vi "MS Updater.vi"(1 "Conveyer Belt Info":T1) -> (0 "Conveyer Belt Info out":T1)   [LabVIEW 2012]
uses:
  Cannon/Cannon Global Data.vi
panel:
  # "s"
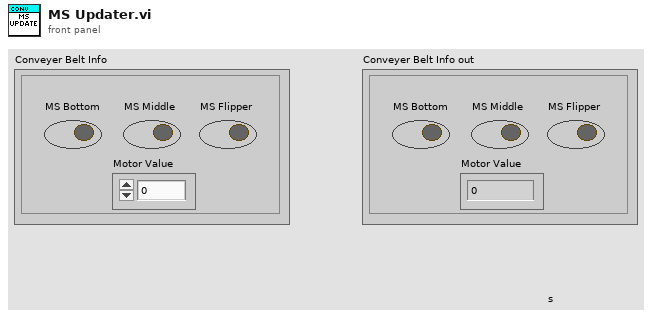
[diagram p1: front panel]
types:
  T1 = cluster{"MS Bottom":bool, "MS Middle":bool, "MS Flipper":bool, "Motor Value":dbl}
  T2 = cluster{"RPM":dbl, "Trigger":bool, "Angle Axis":dbl, "Angle":dbl, "Throttle":dbl, "Slow Angle Change?":bool, "Angle Change?":bool}
  T3 = typedef "WPI_DigitalInputDevRef.ctl" = cluster{"DevStatus":errorcluster, "DIO Channel":T4, "Digital Module":T5}
  T4 = typedef "FPGA_DIOChannel.ctl" = enum8{"DIO 1", "DIO 2", "DIO 3", "DIO 4", "DIO 5", "DIO 6", "DIO 7", "DIO 8", "DIO 9", "DIO 10", "DIO 11", "DIO 12", "DIO 13", "DIO 14", "Invalid"}
  T5 = typedef "FPGA_TypedefDigitalModule.ctl" = enum16{"Digital Module 1", "Digital Module 2"}
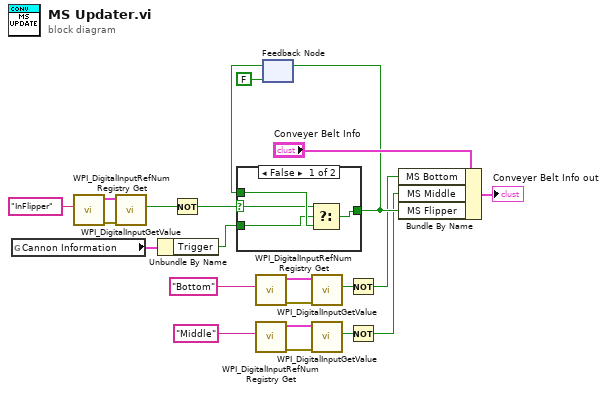
[diagram p0: block diagram]
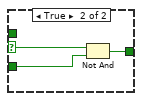
[diagram p2: hidden frame]
diagram:
  n1 = global read "Cannon Global Data.vi" "Cannon Information"() -> (w2:T2)
  n2 = call <vilib>:"WPI_DigitalInputRefNum Registry Get.vi"("refnum name"="InFlipper") -> ("error out"=w16:errorcluster, "DigitalInputDevRef"=w15:T3)  [unwired: 9 in]
  n3 = call <vilib>:"WPI_DigitalInputGetValue.vi"("error in (no error)"=w16, "DigitalInputDevRef"=w15) -> ("Value"=w10:bool)  [unwired: 7 in, 2 out]
  n4 = Unbundle By Name(w2) -> ("Trigger"=w1:bool)
  n5 = Not(x=w10) -> (.not. x?=w7:bool)
  n6 = call <vilib>:"WPI_DigitalInputRefNum Registry Get.vi"("refnum name"="Bottom") -> ("error out"=w17:errorcluster, "DigitalInputDevRef"=w3:T3)  [unwired: 9 in]
  n7 = call <vilib>:"WPI_DigitalInputRefNum Registry Get.vi"("refnum name"="Middle") -> ("error out"=w13:errorcluster, "DigitalInputDevRef"=w14:T3)  [unwired: 9 in]
  n8 = feedback #1(FALSE) -> (w8:bool)
  n9 = case shown="False" w7 {
    selector: w7 -> [w24 w29]
    tunnel: [w26 w28] -> w6
    tunnel: w8 -> [w25 _]
    tunnel: w1 -> [w23 w27]
    frame False {
      n10 = Select(t=w24, s=w23, f=w25) -> (s? t:f=w26:bool)
    }
    frame True {
      n11 = Not And(1:w27, 2:w29) -> (0:w28:bool)
    }
  }
  n12 = feedback-in #1(w6) -> ()
  n13 = call <vilib>:"WPI_DigitalInputGetValue.vi"("error in (no error)"=w17, "DigitalInputDevRef"=w3) -> ("Value"=w12:bool)  [unwired: 7 in, 2 out]
  n14 = call <vilib>:"WPI_DigitalInputGetValue.vi"("error in (no error)"=w13, "DigitalInputDevRef"=w14) -> ("Value"=w11:bool)  [unwired: 7 in, 2 out]
  n15 = Not(x=w12) -> (.not. x?=w4:bool)
  n16 = Not(x=w11) -> (.not. x?=w5:bool)
  n17 = Bundle By Name(cluster="Conveyer Belt Info", "MS Bottom"=w4, "MS Middle"=w5, "MS Flipper"=w6) -> (→"Conveyer Belt Info out":T1)
